vi "setParamsStim.vi"(8 "error in (no error)":errorcluster, 10 "Params":T1={"Mice ID"=[], "ExpType"=[], "Trial Interval"=[], "Pulse Duration"=[], "microL_per_pulse"=[], "Response Interval"=[], "Bad Delay"=[], "Response Period"=[], "liquid_type"="water", "Stimuli"=[], "Rewarded Stimuli"=[]}, 11 "Stimulus in":refnum<class "Stimulus.lvclass">) -> (0 "error out":errorcluster, 3 "Stimulus out":refnum<class "Stimulus.lvclass">)   [LabVIEW 2014, in "Stimulus.lvclass"]
uses:
  Stimulus.lvclass
  Stimulus.lvclass/Stimulus.ctl
  <vilib>/vision/Image Controls.llb/IMAQ Image.ctl
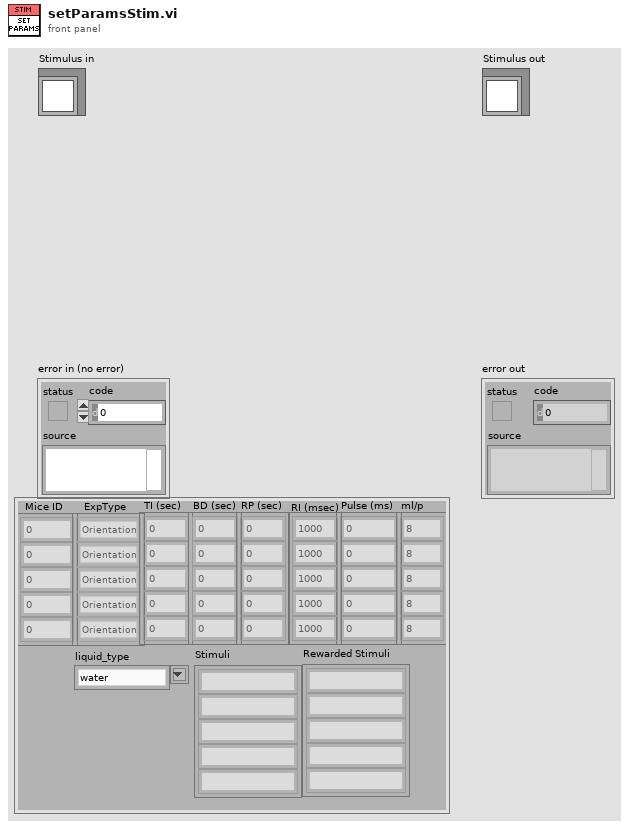
[diagram p1: front panel]
types:
  T1 = cluster{"Mice ID":dbl[], "ExpType":enum16{"Orientation", "Calibrate", "Freerun", "BW"}[], "Trial Interval":dbl[], "Pulse Duration":dbl[], "microL_per_pulse":dbl[], "Response Interval":dbl[], "Bad Delay":dbl[], "Response Period":dbl[], "liquid_type":string, "Stimuli":string[], "Rewarded Stimuli":string[]}
  T2 = typedef "IMAQ Image.ctl" = refnum<image>
  T3 = cluster{"Image":T2, "Window Number (0...15)":i32, "Coordinates (screen)":cluster{"X Position":i32, "Y Position":i32}, "Window name":string, "Time":dbl, "Response \nperiod":dbl, "TI delay":dbl, "Punishment Delay":dbl, "Stim queue":refnum<queue>, "ExpType":enum16{"Orientation", "Calibrate", "Freerun", "BW"}, "Stimuli":string, "Rewarded Stimuli":string, "RI":dbl, "Correct response":bool}
  T4 = cluster{"Image":T2, "Window Number (0...15)":i32, "Coordinates (screen)":cluster{"X Position":i32, "Y Position":i32}, "Window name":string, "Time":dbl, "Response \nperiod":dbl, "TI delay":dbl, "Punishment Delay":dbl, "Stim queue":refnum<queue>, "ExpType":enum16{"Orientation", "Calibrate", "Freerun", "BW"}, "Stimuli":string, "Rewarded Stimuli":string, "RI":dbl, "Correct response":bool}[]
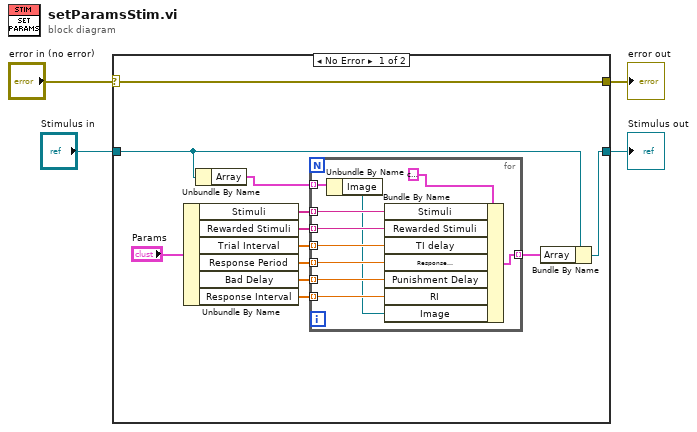
[diagram p0: block diagram]
diagram:
  n1 = case shown="No Error" "error in (no error)" {
    selector: "error in (no error)" -> [w16 w28]
    tunnel: [w16 w28] -> w3
    tunnel: [w7 w27] -> w1
    tunnel: "Stimulus in" -> [w6 w27]
    frame No Error {
      n2 = Unbundle By Name("Params") -> ("Stimuli"=w14:string[], "Rewarded Stimuli"=w9:string[], "Trial Interval"=w10:dbl[], "Response Period"=w11:dbl[], "Bad Delay"=w12:dbl[], "Response Interval"=w13:dbl[])
      n3 = Unbundle By Name(w6) -> ("Array"=w5:T4)
      n4 = for {
        tunnel: w14 -> [w26] mode=indexing
        tunnel: w13 -> [w25] mode=indexing
        tunnel: w12 -> [w24] mode=indexing
        tunnel: w11 -> [w23] mode=indexing
        tunnel: w10 -> [w22] mode=indexing
        tunnel: w9 -> [w21] mode=indexing
        tunnel: [w20] -> w8 mode=indexing
        tunnel: w5 -> [w18] mode=indexing
        n5 = Unbundle By Name(w18) -> ("Image"=w17:T2)
        n6 = Bundle By Name(cluster=T3 {"Image"=refnum, "Window Number (0...15)"=0, "Coordinates (screen)"={"X Position"=0, "Y Position"=0}, "Window name"="", "Time"=0.0, "Response \nperiod"=0.0, "TI delay"=0.0, "Punishment Delay"=0.0, "Stim queue"=refnum, "ExpType"=enum."Orientation", "Stimuli"="", "Rewarded Stimuli"="", "RI"=0.0, "Correct response"=FALSE} ("Cluster"), "Stimuli"=w26, "Rewarded Stimuli"=w21, "TI delay"=w22, "Response \nperiod"=w23, "Punishment Delay"=w24, "RI"=w25, "Image"=w17) -> (w20:T3)
      }
      n7 = Bundle By Name(cluster=w6, "Array"=w8) -> (w7:refnum<class "Stimulus.lvclass">)
    }
    frame Error {
    }
  }
  "error out" <- w3
  "Stimulus out" <- w1
